vi "07 Arrays.vi"() -> ()   [LabVIEW 2019]
panel:
  out "concatenate":i32[](array[numeric])
  out "Matrix":i32[][](array[numeric])
  out "upper part":i32[](array[numeric])
  out "A[4]":i32
  out "Flipped Array":i32[](graph)
  out "Initial Array":i32[](array[numeric])
  # "Hit the Run arrow and see the code execute"
  # "Hit Cmd E to see the diagram (code)"
  # "Vary the array index"
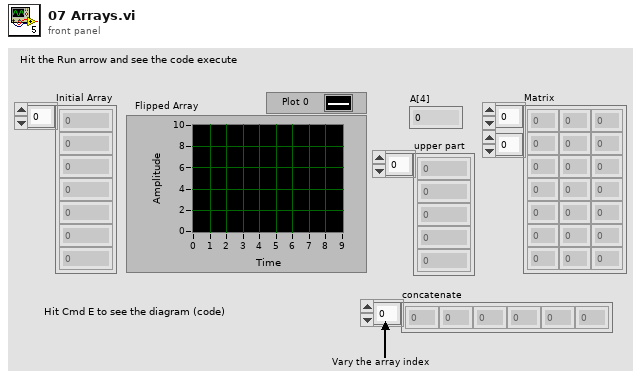
[diagram p1: front panel]
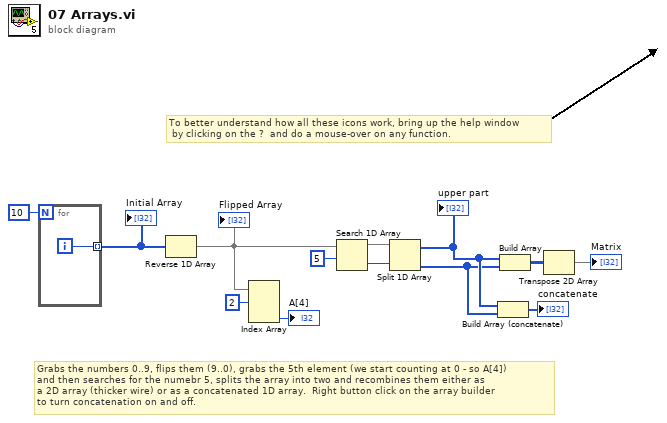
[diagram p0: block diagram]
diagram:
  # "Grabs the numbers 0..9, flips them (9..0), grabs the 5th element (we start counting at 0 - so A[4])\nand then searches for the numebr 5, splits the array into two and recombines them either as\na 2D array (thicker wire) or as a concatenated 1D array.  Right button click on the array builder\nto turn concatenation on and off."
  # "To better understand how all these icons work, bring up the help window\n by clicking on the ?  and do a mouse-over on any function."
  n1 = for {
    N: 10 -> [_]
    tunnel: [w13] -> w11 mode=indexing
    i -> [w13]
  }
  "Initial Array" <- w11
  n2 = Reverse 1D Array(array=w11) -> (reversed array=w7:i32[])
  "Flipped Array" <- w7
  n3 = Index Array(array=w7, index #1=2 ("index")) -> (element #3=→"A[4]":i32)  [unwired: 2 in, 2 out]
  n4 = Search 1D Array(1D array=w7, element=5 ("index")) -> (index of element=w6:i32)  [unwired: 1 in]
  n5 = Split 1D Array(array=w7, index=w6) -> (first subarray=w3:i32[], second subarray=w2:i32[])
  "upper part" <- w3
  n6 = Build Array (concatenate)(w3, w2) -> (→"concatenate":i32[])
  n7 = Build Array(w3, w2) -> (w5:i32[][])
  n8 = Transpose 2D Array(2D array=w5) -> (transposed array=→"Matrix":i32[][])
